vi "measure_current_keithley-2400.vi"(8 "error in (no error)":errorcluster, 11 "VISA resource name":refnum<visa-resource-name>="GPIB1::24::INSTR") -> (0 "error out":errorcluster, 3 "Current":dbl)   [LabVIEW 2016]
uses:
  <instrlib>/Keithley 24XX/Public/Data/Read (Single Point).vi
  <instrlib>/Keithley 24XX/Keithley 24XX.lvlib
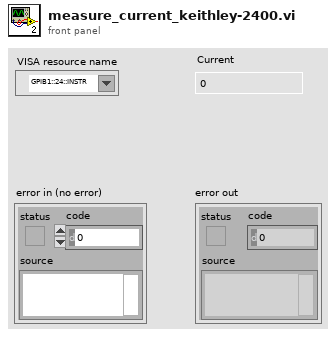
[diagram p1: front panel]
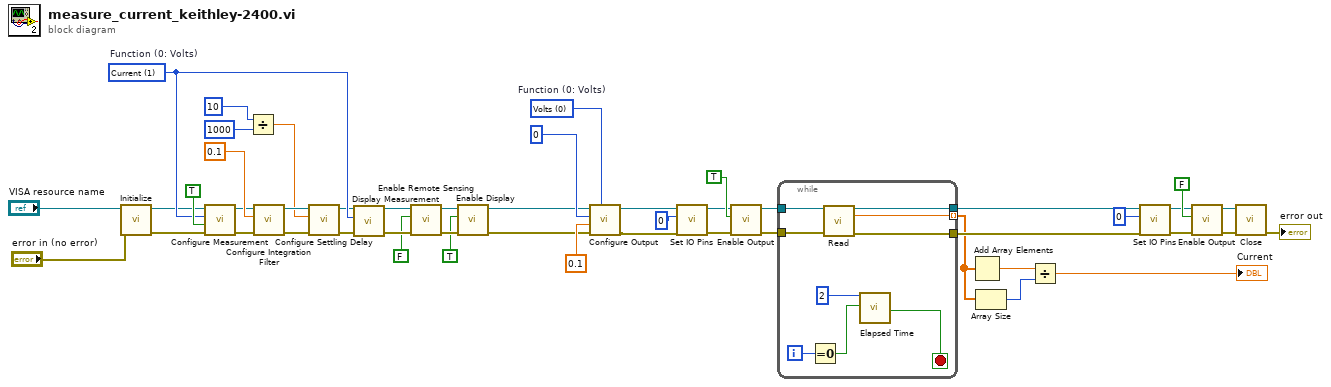
[diagram p0: block diagram]
diagram:
  w16 = u16 0 items=["Volts", "Current", "Resistance"]  # Function (0: Volts)
  w43 = u16 1 items=["Volts", "Current", "Resistance"]  # Function (0: Volts)
  n1 = call <instrlib>:"Initialize.vi"("error in (no error)"="error in (no error)", "VISA resource name"="VISA resource name") -> ("error out"=w33:errorcluster, "VISA resource name out"=w34:refnum<visa-resource-name>)  [unwired: 3 in, 5 out]
  n2 = call <instrlib>:"Configure Measurement.vi"("error in (no error)"=w33, "Enable Auto Range (T:Enable)"=TRUE, "Function (0: Volts)"=w43, "VISA resource name"=w34) -> ("error out"=w36:errorcluster, "VISA resource name out"=w35:refnum<visa-resource-name>)  [unwired: 6 in]
  n3 = Divide(x=10, y=1000) -> (x/y=w42:dbl)
  n4 = call <instrlib>:"Configure Integration Filter.vi"("error in (no error)"=w36, "Measurement Speed (1 PLC)"=0.1, "VISA resource name"=w35) -> ("error out"=w45:errorcluster, "VISA resource name out"=w44:refnum<visa-resource-name>)  [unwired: 7 in]
  n5 = call <instrlib>:"Configure Settling Delay.vi"("error in (no error)"=w45, "Manual Settling Delay (0 sec)"=w42, "VISA resource name"=w44) -> ("error out"=w40:errorcluster, "VISA resource name out"=w39:refnum<visa-resource-name>)  [unwired: 7 in]
  n6 = call <instrlib>:"Display Measurement.vi"("error in (no error)"=w40, "Displayed Measurement (0: Voltage)"=w43, "VISA resource name"=w39) -> ("error out"=w38:errorcluster, "VISA resource name out"=w37:refnum<visa-resource-name>)  [unwired: 7 in]
  n7 = call <instrlib>:"Enable Remote Sensing.vi"("error in (no error)"=w38, "Enable Remote Sensing (T: Enable)"=FALSE, "VISA resource name"=w37) -> ("error out"=w31:errorcluster, "VISA resource name out"=w32:refnum<visa-resource-name>)  [unwired: 7 in]
  n8 = call <instrlib>:"Enable Display.vi"("error in (no error)"=w31, "Enable Display (T: Enable)"=TRUE ("Enable Output (T: Enable)"), "VISA resource name"=w32) -> ("error out"=w3:errorcluster, "VISA resource name out"=w4:refnum<visa-resource-name>)  [unwired: 7 in]
  n9 = call <instrlib>:"Configure Output.vi"("Source Mode  (0: Voltage)"=w16, "error in (no error)"=w3, "Compliance  Level (0.1)"=0.1 ("Compliance  Level"), "Output Level (0)"=0, "VISA resource name"=w4) -> ("error out"=w7:errorcluster, "VISA resource name out"=w8:refnum<visa-resource-name>)  [unwired: 5 in]
  n10 = call <instrlib>:"Set IO Pins.vi"("error in (no error)"=w7, "Output Pattern (0)"=0 ("Numeric"), "VISA resource name"=w8) -> ("error out"=w5:errorcluster, "VISA resource name out"=w6:refnum<visa-resource-name>)  [unwired: 7 in]
  n11 = call <instrlib>:"Enable Output.vi"("error in (no error)"=w5, "Enable Output (T: Enable)"=TRUE ("Output (Off)"), "VISA resource name"=w6) -> ("error out"=w26:errorcluster, "VISA resource name out"=w27:refnum<visa-resource-name>)  [unwired: 7 in]
  n12 = while {
    tunnel: w27 -> [w57]
    tunnel: w26 -> [w56]
    tunnel: [w55] -> w21
    tunnel: [w53] -> w13 mode=indexing
    tunnel: [w49] -> w18
    i -> [w52]
    stop <- w54 stop-if-true
    n13 = Equal To 0?(x=w52) -> (x = 0?=w51:bool)
    n14 = call-poly <instrlib>:"Read.vi"("VISA resource name"=w57, "error in (no error)"=w56) -> ("VISA resource name out"=w55:refnum<visa-resource-name>, "Current"=w53:sgl, "error out"=w49:errorcluster)  [unwired: 7 in, 4 out]
    n15 = call "Elapsed Time"("Time Target (s)"=2, "Reset"=w51) -> ("Time has Elapsed"=w54:bool)  [unwired: 10 in, 7 out]
  }
  n16 = Add Array Elements(numeric array=w13) -> (sum=w14:sgl)
  n17 = Array Size(array=w13) -> (size(s)=w12:i32)
  n18 = Divide(x=w14, y=w12) -> (x/y=→"Current":sgl)
  n19 = call <instrlib>:"Set IO Pins.vi"("error in (no error)"=w18, "Output Pattern (0)"=0, "VISA resource name"=w21) -> ("error out"=w17:errorcluster, "VISA resource name out"=w22:refnum<visa-resource-name>)  [unwired: 7 in]
  n20 = call <instrlib>:"Enable Output.vi"("error in (no error)"=w17, "Enable Output (T: Enable)"=FALSE ("Output (Off)"), "VISA resource name"=w22) -> ("error out"=w24:errorcluster, "VISA resource name out"=w25:refnum<visa-resource-name>)  [unwired: 7 in]
  n21 = call <instrlib>:"Close.vi"("error in (no error)"=w24, "VISA resource name"=w25) -> ("error out"=→"error out":errorcluster)  [unwired: 9 in]
